vi "NInstrSim_ConfigureVDCRange.appendData2Variant.vi"(0 "initData":variant, 2 "DC Voltage Range (1:10 VDC)":u16(ring)=1 items=["0:1 VDC", "0:10 VDC", "0:100 VDC"], 5 "error in (no error)":errorcluster) -> (14 "dup initData":variant, 19 "error out":errorcluster)   [LabVIEW 2009, in "HB_Device_Examples.lvlib" / "NInstrSim_ConfigureVDCRange.lvclass"]
doc: "Append initialize data to variant."
uses:
  NInstrSim_ConfigureVDCRange.lvclass
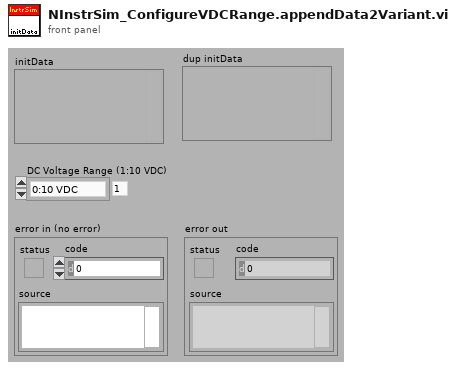
[diagram p1: front panel]
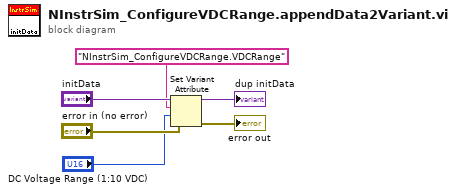
[diagram p0: block diagram]
diagram:
  n1 = Set Variant Attribute(Variant="initData", name="NInstrSim_ConfigureVDCRange.VDCRange", value="DC Voltage Range (1:10 VDC)", error in="error in (no error)") -> (Variant out=→"dup initData":variant, error out=→"error out":errorcluster)  [unwired: 1 out]
